vi "Axis_Point Table.vi"(7 "Enum":T2(ring)=enum."WritePoint", 8 "error In":errorcluster, 9 "PointIn":string[][](array[string]), 10 "AxisData":T3={"AxisName"="Axis_X", "Accel"=0.0, "Deaccel"=0.0, "Speed"=0.0, "Sramp"=0.0}, 11 "AxisIndex":i32) -> (0 "error Out":errorcluster, 2 "AxisSpeed Basic":T1(array[cluster]), 3 "RobotPoint":string[][](table))   [LabVIEW 2019]
uses:
  9ad018fe-fe3d-4d70-b9e6-1139023f1b05.vi
  9f834300-6493-4986-9df7-de3f3f8a56bc.vi
  LLB/Commonly VI/Main Glb.vi
  <vilib>/Utility/config.llb/Read Key (String).vi
  <vilib>/JDP Science/JSONtext/JSON text to Variant.vi
  <vilib>/JDP Science/JSONtext/Variant to JSON Text.vi
  <vilib>/Utility/config.llb/Write Key (String).vi
  LLB/Commonly VI.lvlib
  <vilib>/Utility/config.llb/NI_LVConfig.lvlib
panel:
  in  "AxisSpeed Basic 2":T1(array[cluster])=[{"AxisName"="Axis_X", "Accel"=0.5, "Deaccel"=0.5, "Speed"=200.0, "Sramp"=0.5}, {"AxisName"="Axis_Y", "Accel"=0.5, "Deaccel"=0.5, "Speed"=200.0, "Sramp"=0.5}, {"AxisName"="Axis_Z", "Accel"=0.5, "Deaccel"=0.5, "Speed"=200.0, "Sramp"=0.5}, {"AxisName"="Axis_U", "Accel"=0.0, "Deaccel"=0.0, "Speed"=0.0, "Sramp"=0.0}]
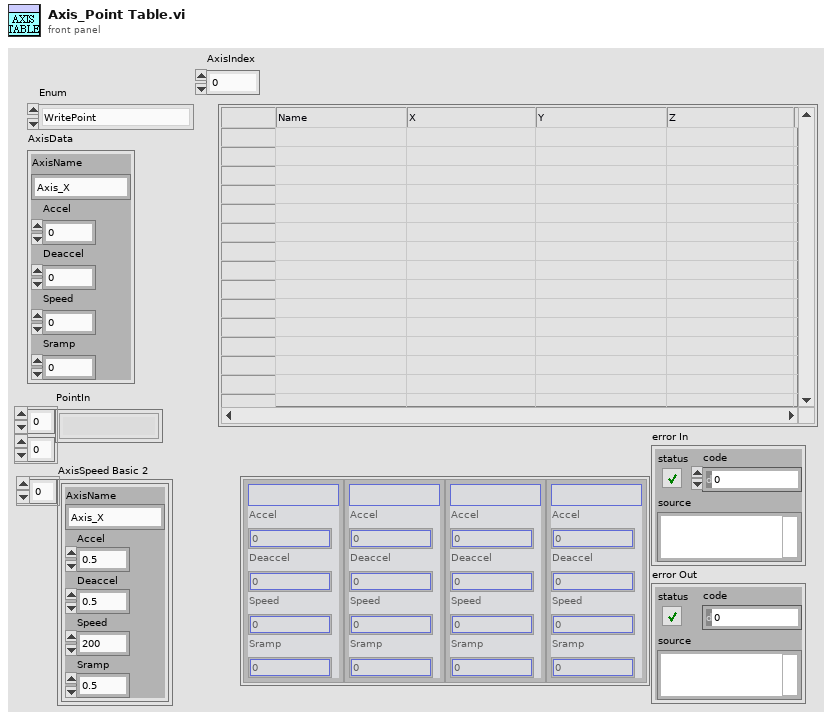
[diagram p1: front panel]
types:
  T1 = cluster{"AxisName":string, "Accel":dbl, "Deaccel":dbl, "Speed":dbl, "Sramp":dbl}[]
  T2 = enum16{"Initial", "Load", "Save", "Read", "WriteSpeed", "WritePoint"}
  T3 = cluster{"AxisName":string, "Accel":dbl, "Deaccel":dbl, "Speed":dbl, "Sramp":dbl}
  T4 = cluster{"AxisSpeed":cluster{"Axis":cluster{"AxisName":string, "Accel":dbl, "Deaccel":dbl, "Speed":dbl, "Sramp":dbl}[]}, "Point":string[][]}
  T5 = typedef "NI_LVConfig.lvlib/Config Data RefNum.ctl" = refnum<k1>
  T6 = cluster{"AxisSpeed Basic":cluster{"AxisName":string, "Accel":dbl, "Deaccel":dbl, "Speed":dbl, "Sramp":dbl}[]}
  T7 = cluster{"Axis":cluster{"AxisName":string, "Accel":dbl, "Deaccel":dbl, "Speed":dbl, "Sramp":dbl}[]}
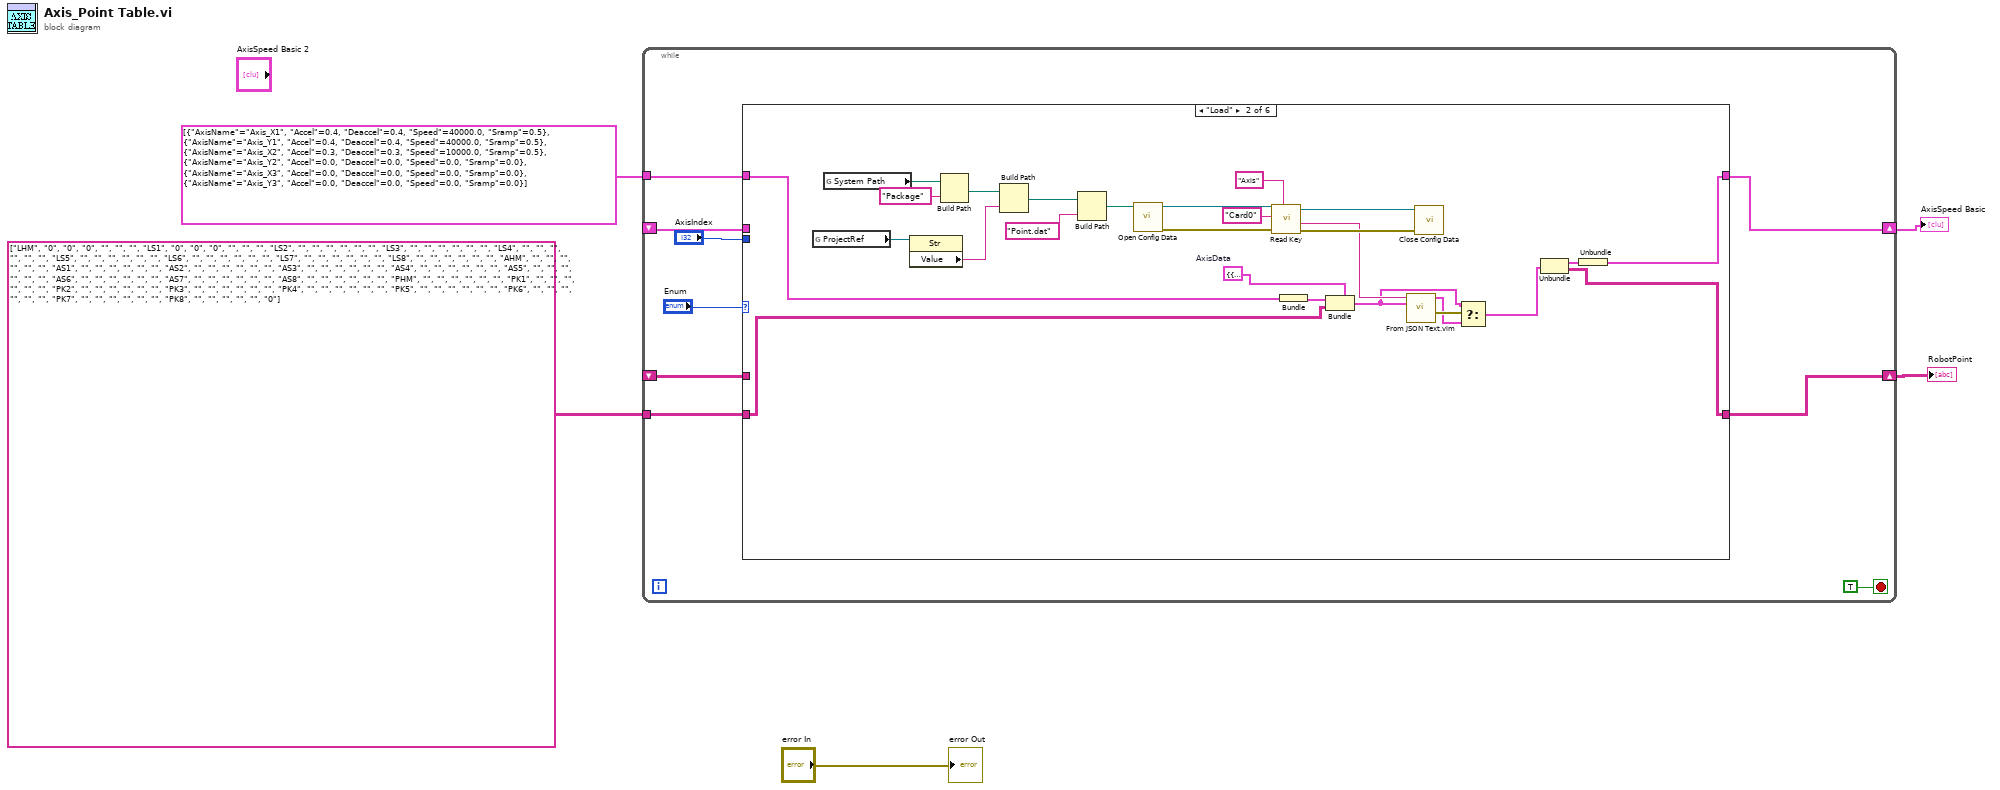
[diagram p0: block diagram]
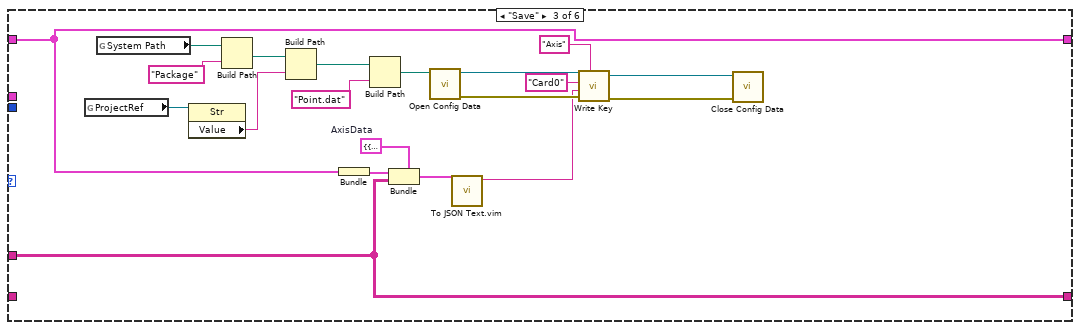
[diagram p3: hidden frame]
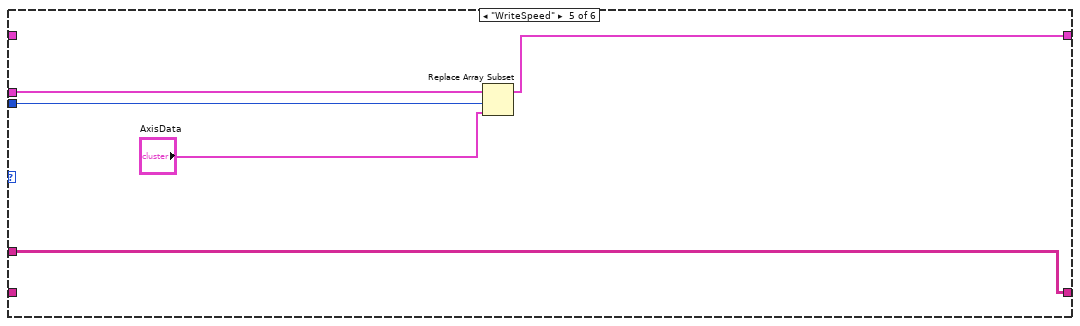
[diagram p5: hidden frame]
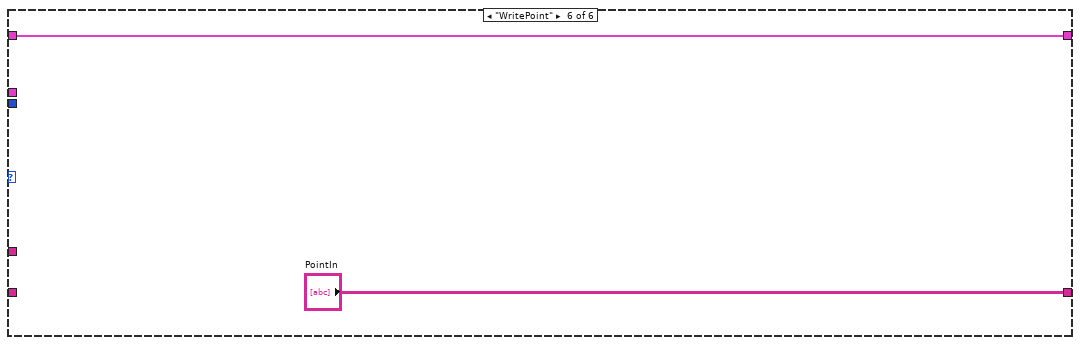
[diagram p6: hidden frame]
diagram:
  n1 = while {
    shift-right: [w12] -> w2
    shift-left: _ -> [w13]
    tunnel: T1 [{"AxisName"="Axis_X1", "Accel"=0.4, "Deaccel"=0.4, "Speed"=40000.0, "Sramp"=0.5}, {"AxisName"="Axis_Y1", "Accel"=0.4, "Deaccel"=0.4, "Speed"=40000.0, "Sramp"=0.5}, {"AxisName"="Axis_X2", "Accel"=0.3, "Deaccel"=0.3, "Speed"=10000.0, "Sramp"=0.5}, {"AxisName"="Axis_Y2", "Accel"=0.0, "Deaccel"=0.0, "Speed"=0.0, "Sramp"=0.0}, {"AxisName"="Axis_X3", "Accel"=0.0, "Deaccel"=0.0, "Speed"=0.0, "Sramp"=0.0}, {"AxisName"="Axis_Y3", "Accel"=0.0, "Deaccel"=0.0, "Speed"=0.0, "Sramp"=0.0}] ("AxisSpeed Basic") -> [w11]
    tunnel: string[][] [["LHM", "0", "0", "0", "", "", ""], ["LS1", "0", "0", "0", "", "", ""], ["LS2", "", "", "", "", "", ""], ["LS3", "", "", "", "", "", ""], ["LS4", "", "", "", "", "", ""], ["LS5", "", "", "", "", "", ""], ["LS6", "", "", "", "", "", ""], ["LS7", "", "", "", "", "", ""], ["LS8", "", "", "", "", "", ""], ["AHM", "", "", "", "", "", ""], ["AS1", "", "", "", "", "", ""], ["AS2", "", "", "", "", "", ""], ["AS3", "", "", "", "", "", ""], ["AS4", "", "", "", "", "", ""], ["AS5", "", "", "", "", "", ""], ["AS6", "", "", "", "", "", ""], ["AS7", "", "", "", "", "", ""], ["AS8", "", "", "", "", "", ""], ["PHM", "", "", "", "", "", ""], ["PK1", "", "", "", "", "", ""], ["PK2", "", "", "", "", "", ""], ["PK3", "", "", "", "", "", ""], ["PK4", "", "", "", "", "", ""], ["PK5", "", "", "", "", "", ""], ["PK6", "", "", "", "", "", ""], ["PK7", "", "", "", "", "", ""], ["PK8", "", "", "", "", "", "0"]] -> [w10]
    shift-right: [w9] -> w3
    shift-left: _ -> [w7]
    stop <- TRUE stop-if-true
    n2 = case shown="\"Load\"" "Enum" {
      tunnel: w13 -> [_ _ _ w64 w69 _]
      tunnel: [w16 w25 w47 w64 w68 w71] -> w12
      tunnel: w11 -> [w16 w29 w47 _ _ w71]
      tunnel: w10 -> [w15 w27 _ _ _ _]
      tunnel: [w15 w24 w43 w63 w67 "PointIn"] -> w9
      tunnel: w7 -> [_ _ w43 w63 w67 _]
      tunnel: "AxisIndex" -> [_ _ _ _ w65 _]
      frame "Initial", Default {
      }
      frame "Load" {
        w23 = T4 {"AxisSpeed"={"Axis"=[]}, "Point"=[]}  # AxisData
        n3 = global read "Main Glb.vi" "ProjectRef"() -> (w39:refnum<vi>)
        n4 = global read "Main Glb.vi" "System Path"() -> (w42:path)
        n5 = property class="Str"(reference=w39) -> ("Value"=w21:string)  [unwired: 1 in, 2 out]
        n6 = Build Path(base path=w42, name or relative path="Package") -> (appended path=w40:path)
        n7 = Build Path(base path=w40, name or relative path=w21) -> (appended path=w38:path)
        n8 = Build Path(base path=w38, name or relative path="Point.dat") -> (appended path=w36:path)
        n9 = call <vilib>:"Open Config Data.vi"("configuration file path"=w36) -> ("error out"=w34:errorcluster, "refnum"=w35:T5)  [unwired: 8 in, 1 out]
        n10 = call-poly <vilib>:"Read Key.vi"("section"="Axis", "error in (no error)"=w34, "key"="Card0", "refnum"=w35) -> ("error out"=w30:errorcluster, "value"=w22:string, "refnum out"=w31:T5)  [unwired: 4 in, 1 out]
        n11 = Bundle("AxisSpeed Basic"=w29) -> (w28:T6)  [unwired: 1 in]
        n12 = Bundle(cluster=w23, "AxisSpeed"=w28, "Point"=w27) -> (w17:T4)
        n13 = call "From JSON Text.vim"("Data Type and Default Value"=w17, "JSON"=w22) -> ("error out"=w20:errorcluster, "Data out"=w19:T4)  [unwired: 8 in]
        n14 = call <vilib>:"Close Config Data.vi"("error in (no error)"=w30, "refnum"=w31) -> ()  [unwired: 8 in, 2 out]
        n15 = Select(t=w17, s=w20, f=w19) -> (s? t:f=w18:T4)
        n16 = Unbundle(w18) -> ("AxisSpeed"=w26:T7, "Point"=w24:string[][])
        n17 = Unbundle(w26) -> ("Axis"=w25:T1)
      }
      frame "Save" {
        w48 = T4 {"AxisSpeed"={"Axis"=[]}, "Point"=[]}  # AxisData
        n18 = global read "Main Glb.vi" "ProjectRef"() -> (w59:refnum<vi>)
        n19 = global read "Main Glb.vi" "System Path"() -> (w62:path)
        n20 = property class="Str"(reference=w59) -> ("Value"=w44:string)  [unwired: 1 in, 2 out]
        n21 = Build Path(base path=w62, name or relative path="Package") -> (appended path=w60:path)
        n22 = Build Path(base path=w60, name or relative path=w44) -> (appended path=w58:path)
        n23 = Bundle("AxisSpeed Basic"=w47) -> (w49:T6)  [unwired: 1 in]
        n24 = Build Path(base path=w58, name or relative path="Point.dat") -> (appended path=w56:path)
        n25 = Bundle(cluster=w48, "AxisSpeed"=w49, "Point"=w43) -> (w46:T4)
        n26 = call <vilib>:"Open Config Data.vi"("configuration file path"=w56) -> ("error out"=w54:errorcluster, "refnum"=w55:T5)  [unwired: 8 in, 1 out]
        n27 = call "To JSON Text.vim"("Anything"=w46) -> ("<JSON>"=w45:string)  [unwired: 9 in, 1 out]
        n28 = call-poly <vilib>:"Write Key.vi"("section"="Axis", "error in (no error)"=w54, "value"=w45, "key"="Card0", "refnum"=w55) -> ("error out"=w50:errorcluster, "refnum out"=w51:T5)  [unwired: 4 in, 1 out]
        n29 = call <vilib>:"Close Config Data.vi"("error in (no error)"=w50, "refnum"=w51) -> ()  [unwired: 8 in, 2 out]
      }
      frame "Read" {
      }
      frame "WriteSpeed" {
        n30 = Replace Array Subset(array=w69, new element="AxisData", index=w65) -> (w68:T1)
      }
      frame "WritePoint" {
      }
    }
  }
  "RobotPoint" <- w3
  "AxisSpeed Basic" <- w2
  "error Out" <- "error In"
